vi "ICC4C_Analog_Control_Tester_From_CSV_Importer_Template.vi"() -> ()   [LabVIEW 2021]
uses:
  <vilib>/DAQmx/write.llb/DAQmx Write (Analog 1D DBL NChan 1Samp).vi
  <vilib>/DAQmx/create/channels.llb/DAQmx Create Channel (AO-Voltage-Basic).vi
  <vilib>/DAQmx/miscellaneous.llb/DAQmx Fill In Error Info.vi
panel:
  out "ICC4C 0":dbl
  out "current mA":dbl
  in  "mA Step Size":dbl
  in  "Y1 (-10-10V)":dbl
  in  "X1 (-10-10V)":dbl
  out "Raw  Inner Loop Iternation":i32
  out "Andor_V":dbl
  out "Trigger_Phase_Iterations":i32
  in  "Delay (ADDS 3ms)":i32
  in  "ICC4C 3 (0-10V)":dbl
  in  "ICC4C 2 (0-10V)":dbl
  in  "ICC4C 1 (0-10V)":dbl
  in  "Y2 (-10-10V)":dbl
  in  "X2 (-10-10V)":dbl
  in  "Continue Cycle?":bool
  out "Full Cycles":i32
  out "Mirror_Phase_Iterations":i32
  out "Y1 (-10-10V)":dbl format="%_6g"
  out "X1 (-10-10V)":dbl format="%_6g"
  in  "Blanking (0-10v)":dbl=10.0
  in  "561 (0-10v)":dbl
  in  "514 (0-10v)":dbl
  in  "488 (0-10v)":dbl
  in  "445 (0-10v)":dbl
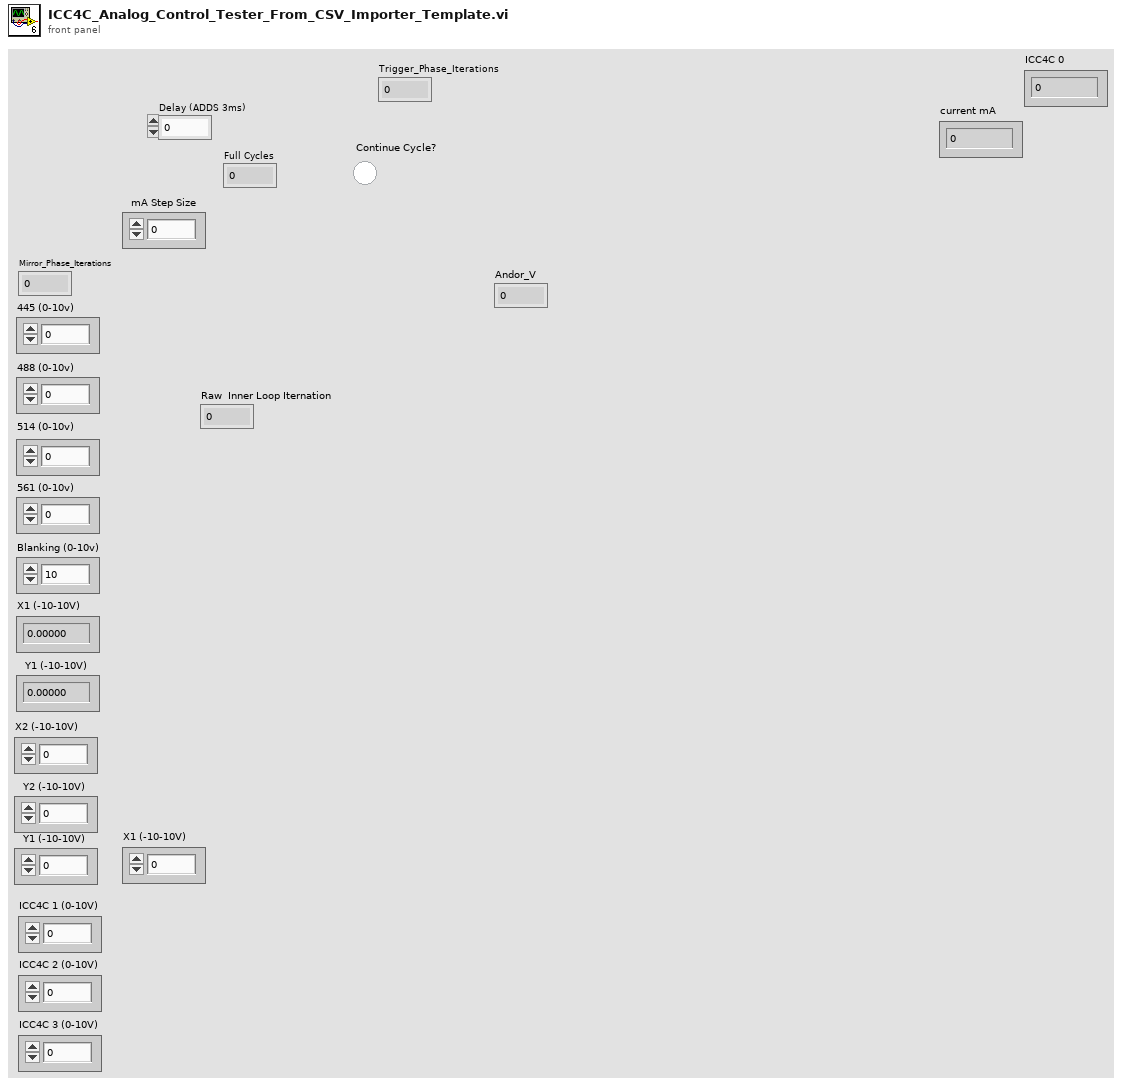
[diagram p1: front panel]
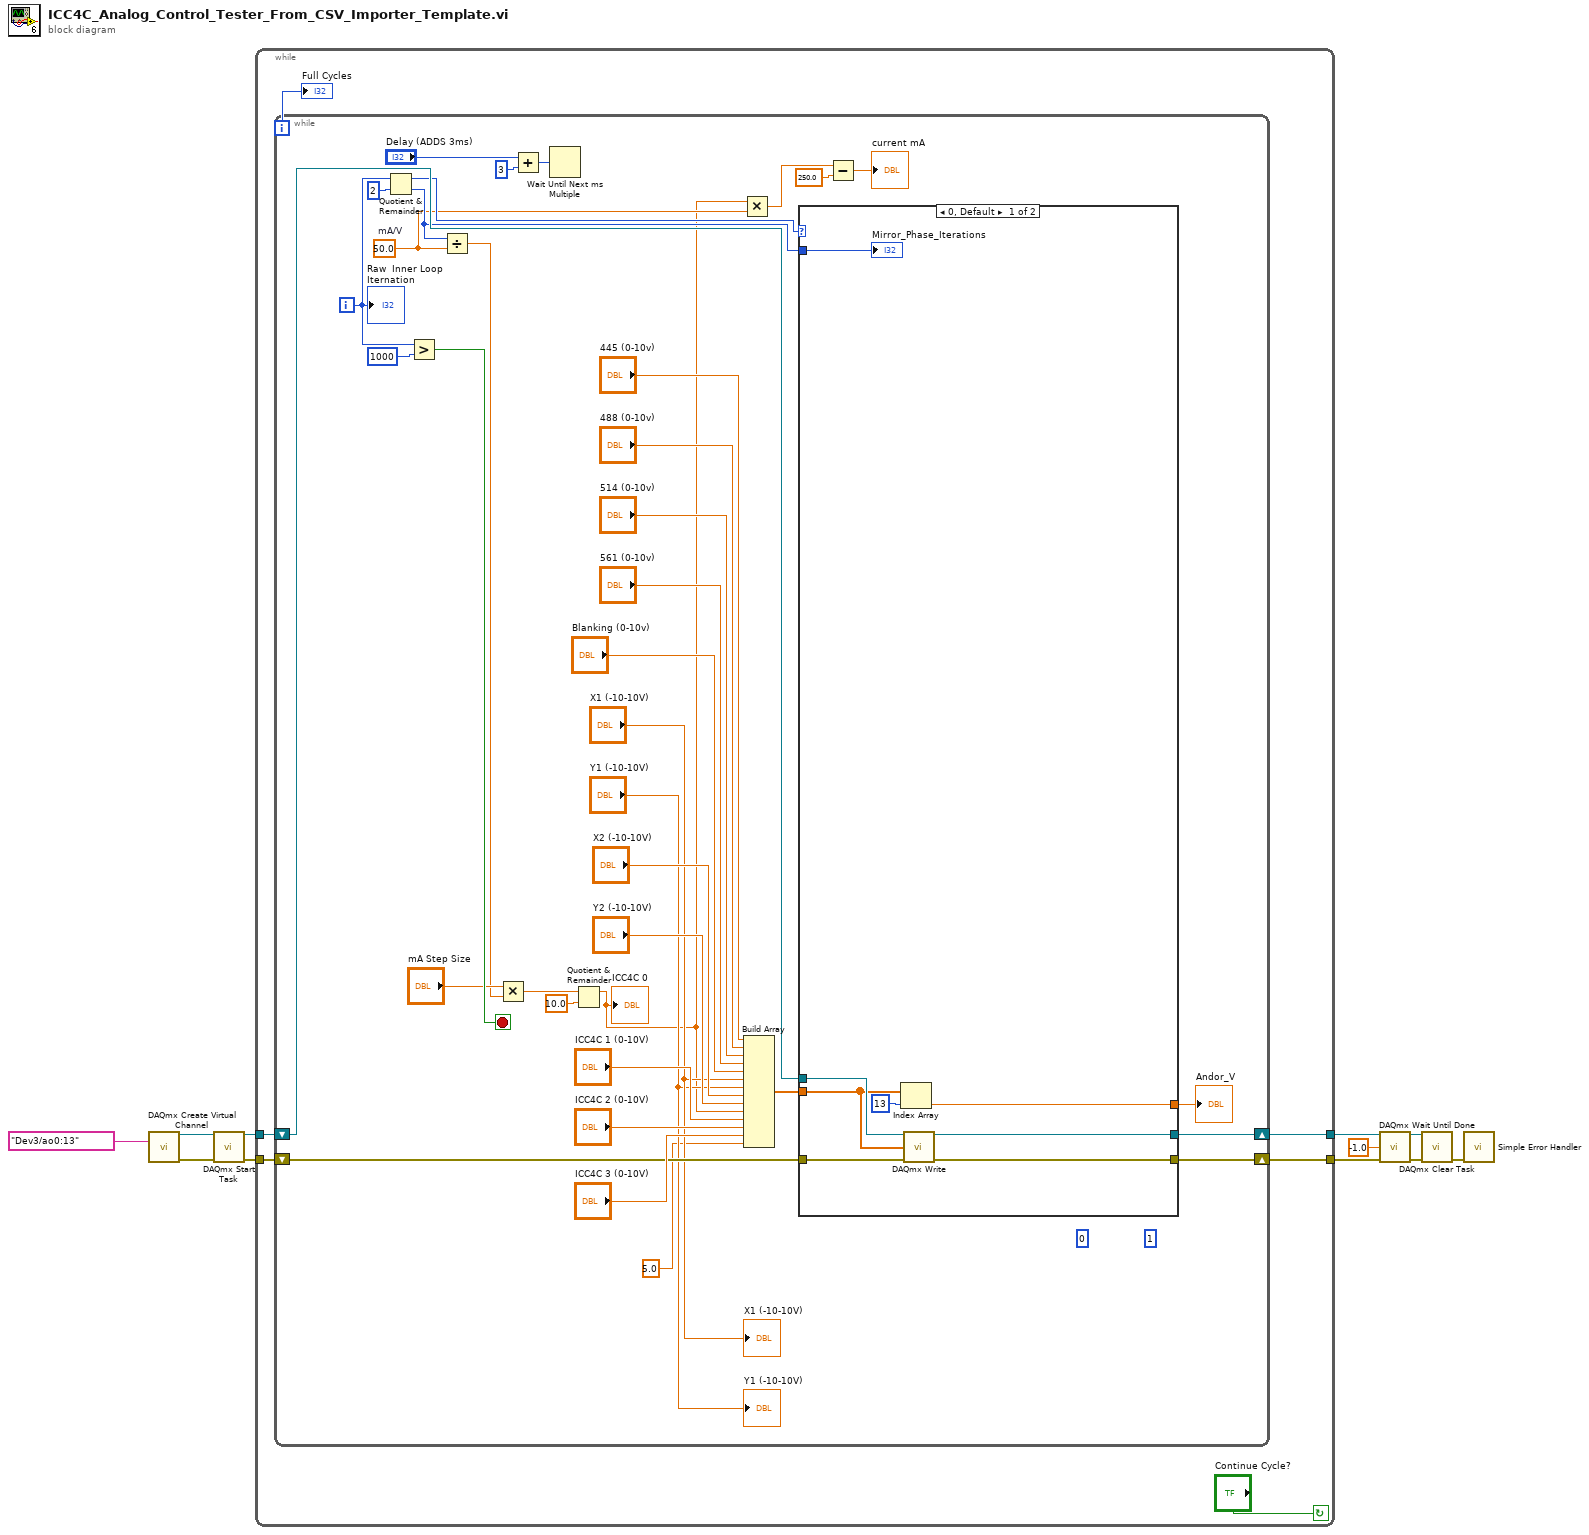
[diagram p0: block diagram]
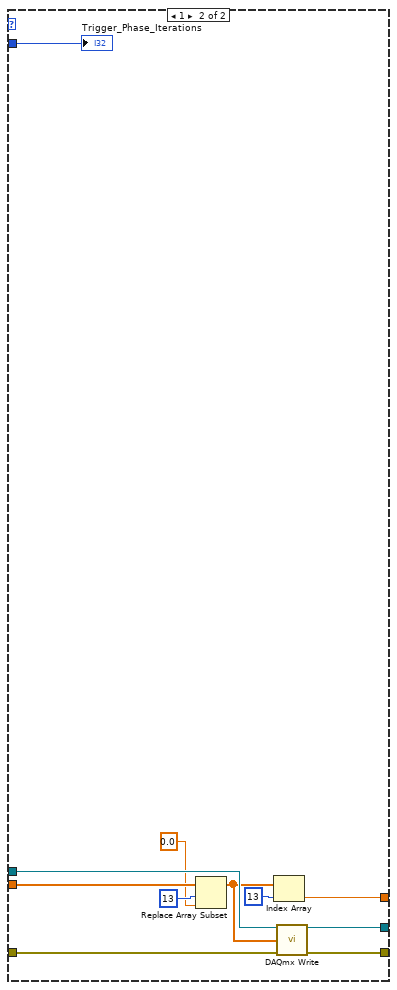
[diagram p2: hidden frame]
diagram:
  n1 = call-poly <vilib>:"DAQmx Create Virtual Channel.vi"("physical channels"=tag "Dev3/ao0:13") -> ("task out"=w4:refnum<k21>, "error out"=w3:errorcluster)  [unwired: 13 in]
  n2 = call <vilib>:"DAQmx Start Task.vi"("task/channels in"=w4, "error in"=w3) -> ("task out"=w2:refnum<k21>, "error out"=w1:errorcluster)  [unwired: 12 in]
  n3 = while {
    tunnel: [w14] -> w7
    tunnel: [w13] -> w6
    tunnel: w2 -> [w16]
    tunnel: w1 -> [w15]
    i -> [w17]
    stop <- "Continue Cycle?" continue-if-true
    n4 = while {
      shift-right: [w42] -> w14
      shift-left: w16 -> [w40]
      shift-right: [w43] -> w13
      shift-left: w15 -> [w39]
      i -> [w31]
      stop <- w29 stop-if-true
      w21 = 50.0  # mA/V
      (unwired) 0
      (unwired) 1
      n5 = Quotient & Remainder(x=w31, y=2) -> (x-y*floor(x/y)=w32:i32, floor(x/y)=w27:i32)
      n6 = Greater?(x=w31, y=1000) -> (0:w29:bool)
      n7 = Divide(x=w27, y=w21) -> (x/y=w26:dbl)
      n8 = Multiply(x="mA Step Size", y=w26) -> (x*y=w23:dbl)
      n9 = Add(x="Delay (ADDS 3ms)", y=3) -> (x+y=w35:i32)
      n10 = Wait Until Next ms Multiple(millisecond multiple=w35) -> ()  [unwired: 1 out]
      n11 = Quotient & Remainder(x=w23, y=10.0) -> (x-y*floor(x/y)=w19:dbl)  [unwired: 1 out]
      "ICC4C 0" <- w19
      n12 = Multiply(x=w19, y=w21) -> (x*y=w20:dbl)
      n13 = Build Array("445 (0-10v)", "488 (0-10v)", "514 (0-10v)", "561 (0-10v)", "Blanking (0-10v)", "X1 (-10-10V)", "Y1 (-10-10V)", "X2 (-10-10V)", "Y2 (-10-10V)", w19, "ICC4C 1 (0-10V)", "ICC4C 2 (0-10V)", "ICC4C 3 (0-10V)", 5.0) -> (w44:dbl[])
      n14 = case shown="0, Default" w32 {
        tunnel: w40 -> [w62 w73]
        tunnel: [w59 w72] -> w42
        tunnel: w39 -> [w61 w71]
        tunnel: [w60 w67] -> w43
        tunnel: w44 -> [w58 w70]
        tunnel: w27 -> [w55 w68]
        tunnel: [w56 w64] -> w38
        frame 0, Default {
          n15 = Index Array(array=w58, index=13) -> (element=w56:dbl)
          n16 = call-poly <vilib>:"DAQmx Write.vi"("task/channels in"=w62, "data"=w58, "error in"=w61) -> ("task out"=w59:refnum<k21>, "error out"=w60:errorcluster)  [unwired: 10 in, 1 out]
          "Mirror_Phase_Iterations" <- w55
        }
        frame 1 {
          n17 = Replace Array Subset(array=w70, new element=0.0, index=13) -> (w65:dbl[])
          n18 = Index Array(array=w65, index=13) -> (element=w64:dbl)
          n19 = call-poly <vilib>:"DAQmx Write.vi"("task/channels in"=w73, "data"=w65, "error in"=w71) -> ("task out"=w72:refnum<k21>, "error out"=w67:errorcluster)  [unwired: 10 in, 1 out]
          "Trigger_Phase_Iterations" <- w68
        }
      }
      "Andor_V" <- w38
      n20 = Subtract(x=w20, y=250.0) -> (x-y=→"current mA":dbl)
      "X1 (-10-10V)" <- "X1 (-10-10V)"
      "Y1 (-10-10V)" <- "Y1 (-10-10V)"
      "Raw  Inner Loop Iternation" <- w31
    }
    "Full Cycles" <- w17
  }
  n21 = call <vilib>:"DAQmx Wait Until Done.vi"("task/channels in"=w7, "timeout (sec)"=-1.0, "error in"=w6) -> ("task out"=w10:refnum<k21>, "error out"=w9:errorcluster)  [unwired: 11 in]
  n22 = call <vilib>:"DAQmx Clear Task.vi"("task in"=w10, "error in"=w9) -> ("error out"=w11:errorcluster)  [unwired: 13 in]
  n23 = call <vilib>:"Simple Error Handler.vi"("error in (no error)"=w11) -> ()  [unwired: 4 in, 5 out]
